vi "Globals.vi"() -> ()   [LabVIEW 2025, in "MCP Demo Application.lvlib"]
uses:
  MCP Demo Application.lvlib
panel:
  in  "FFT Graph Refnum":refnum<vi>
  in  "Chart Refnum":refnum<vi>
  in  "stop":bool
  in  "FFTs":waveform(dbl)[](array[waveform])
  in  "waveforms":waveform(dbl)[](array[waveform])
  in  "Frequency":dbl
  in  "Amplitude":dbl
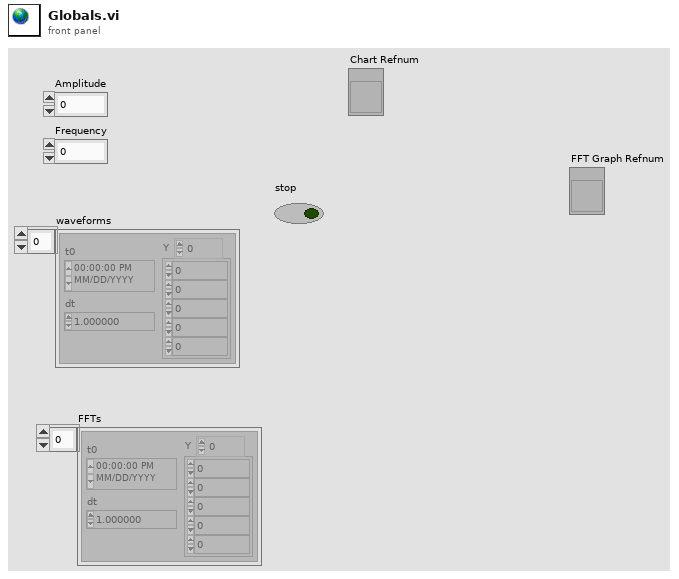
[diagram p1: front panel]
diagram:
